vi "PCert-ConfigPageNF-InRequests.vi"(8 "error in (no error)":errorcluster, 11 "ERP-ConfigPageNF in":refnum<class "PCert-ConfigPageNF.lvclass">) -> (0 "error out":errorcluster, 2 "Incoming Requests":refnum<event-registration>, 3 "ERP-ConfigPageNF out":refnum<class "PCert-ConfigPageNF.lvclass">)   [LabVIEW 2013, in "PCert-ConfigPageNF.lvclass"]
uses:
  PCert-ConfigPageNF.lvclass
  ftw-dataflow/Actor/src/Message/Request/FTW-Message-IncomingRequest.lvclass
  PCert-ConfigPageNF.lvclass/PCert-ConfigPageNF.ctl
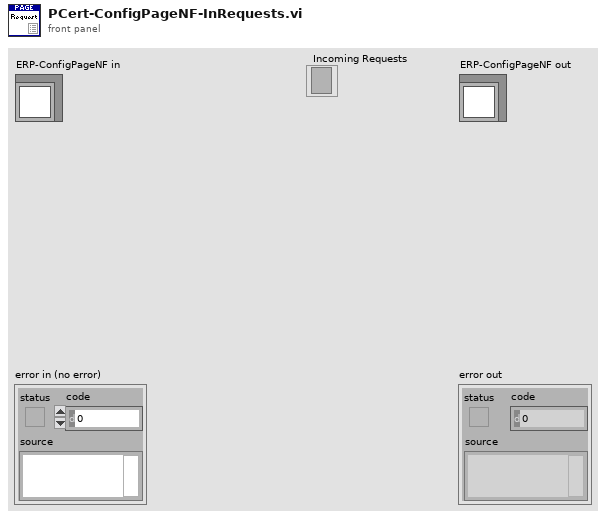
[diagram p1: front panel]
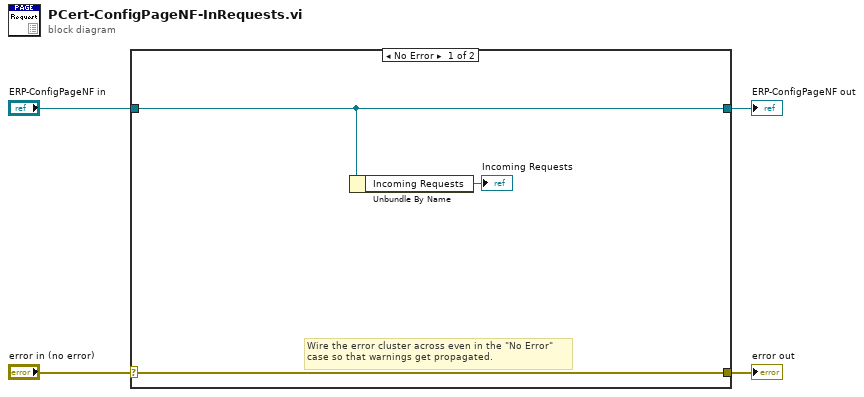
[diagram p0: block diagram]
diagram:
  n1 = case shown="No Error" "error in (no error)" {
    selector: "error in (no error)" -> [w7 w9]
    tunnel: [w7 w9] -> w3
    tunnel: [w6 w8] -> w1
    tunnel: "ERP-ConfigPageNF in" -> [w6 w8]
    frame No Error {
      # "Wire the error cluster across even in the \"No Error\"\ncase so that warnings get propagated."
      n2 = Unbundle By Name(w6) -> ("Incoming Requests"=→"Incoming Requests":refnum<event-registration>)
    }
    frame Error {
    }
  }
  "error out" <- w3
  "ERP-ConfigPageNF out" <- w1
